vi "Ring-Add Prompt.vi"(0 "Ring in":refnum<vi>, 5 "strings":string[](array[string]), 9 "Prompt":string) -> (4 "Ring out":refnum<vi>)   [LabVIEW 2020]
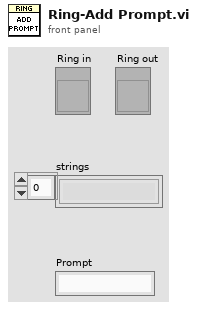
[diagram p1: front panel]
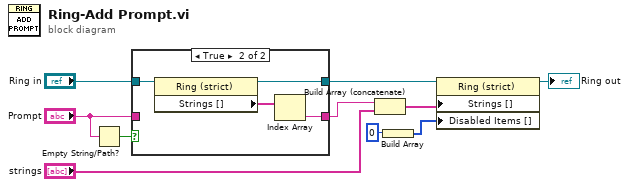
[diagram p0: block diagram]
diagram:
  n1 = Empty String/Path?(string/path="Prompt") -> (empty?=w3:bool)
  n2 = case shown="True" w3 {
    tunnel: "Prompt" -> [w12 _]
    tunnel: [w12 w13] -> w5
    tunnel: "Ring in" -> [w11 w16]
    tunnel: [w11 w15] -> w1
    frame False {
    }
    frame True {
      n3 = property on="Property Node" class="Ring (strict)"(reference=w16) -> (reference out=w15:refnum<vi>, "Strings []"=w14:string[])  [unwired: 1 in, 1 out]
      n4 = Index Array(array=w14) -> (element=w13:string)  [unwired: 1 in]
    }
  }
  n5 = Build Array (concatenate)(w5, "strings") -> (w9:string[])
  n6 = Build Array(0) -> (w7:i32[])
  n7 = property on="Property Node" class="Ring (strict)"(reference=w1, "Strings []"=w9, "Disabled Items []"=w7) -> (reference out=→"Ring out":refnum<vi>)  [unwired: 1 in, 1 out]
